vi "standard deviation2015.vi"() -> ()   [LabVIEW 2015]
uses:
  <vilib>/Analysis/NI_AALBase.lvlib
  <vilib>/Utility/file.llb/Read Delimited Spreadsheet (DBL).vi
panel:
  out "Prepared by \nthe project":string
  out "Data":dbl[][](array[numeric])
  out "Standard Deviation":dbl
  in  "Measurement file \nwith extension Txt":path
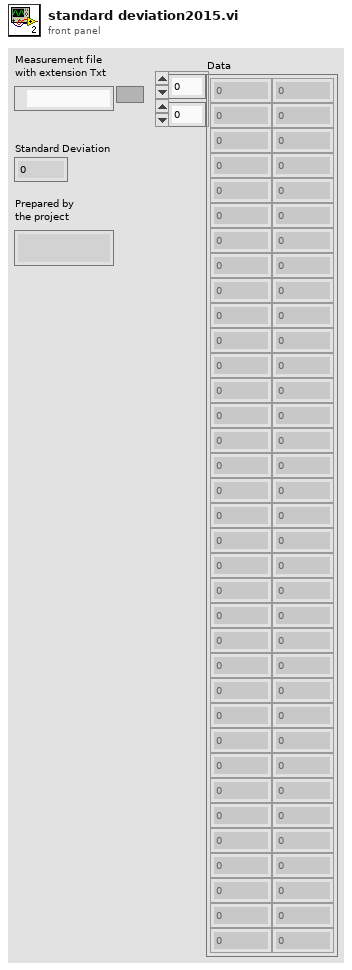
[diagram p1: front panel]
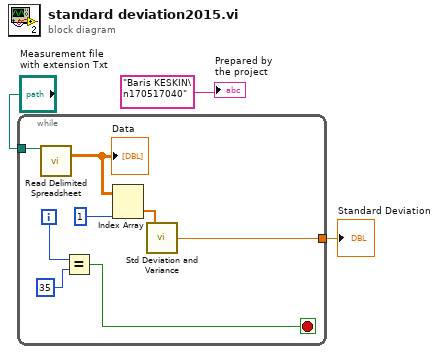
[diagram p0: block diagram]
diagram:
  n1 = while {
    tunnel: "Measurement file \nwith extension Txt" -> [w11]
    tunnel: [w8] -> w2
    i -> [w7]
    stop <- w6 stop-if-true
    n2 = call-poly <vilib>:"Read Delimited Spreadsheet.vi"("file path (dialog if empty)"=w11) -> ("all rows"=w10:dbl[][])  [unwired: 9 in, 5 out]
    "Data" <- w10
    n3 = Equal?(x=w7, y=35) -> (x = y?=w6:bool)
    n4 = Index Array(array=w10, index (col)=1 ("disabled index (col)")) -> (element=w9:dbl[])  [unwired: 1 in]
    n5 = call <vilib>:"Std Deviation and Variance.vi"("X"=w9) -> ("standard deviation"=w8:dbl)  [unwired: 1 in, 2 out]
  }
  "Standard Deviation" <- w2
  "Prepared by \nthe project" <- "Baris KESKIN\n170517040"
